vi "Ex 07 - C-Scan.vi"() -> ()   [LabVIEW 2026]
uses:
  <instrlib>/MicroPulse/Public/Data/Datatypes/MP - data formatting.ctl
  <instrlib>/MicroPulse/Public/Data/Datatypes/MP - amplitude reporting mode.ctl
  <instrlib>/MicroPulse/Public/Data/Datatypes/MP - averaging.ctl
  <instrlib>/MicroPulse/Public/Data/Datatypes/MP - transmit parameters.ctl
  <instrlib>/MicroPulse/Public/Data/Datatypes/MP - pulser voltage.ctl
  <instrlib>/MicroPulse/Public/Data/Datatypes/MP - pulse damping.ctl
  <instrlib>/MicroPulse/Public/Data/Datatypes/MP - test parameters.ctl
  <instrlib>/MicroPulse/Public/Data/Datatypes/MP - receive parameters.ctl
  <instrlib>/MicroPulse/Public/Data/Datatypes/MP - display gate.ctl
  <instrlib>/MicroPulse/Public/Data/Datatypes/MP - waveform type.ctl
  <instrlib>/MicroPulse/Public/Data/Datatypes/MP - analogue filter.ctl
  <instrlib>/MicroPulse/Public/Data/Datatypes/MP - frequency filter.ctl
  <instrlib>/MicroPulse/Public/Data/Datatypes/MP - digital filtering.ctl
  <instrlib>/MicroPulse/Public/Data/Datatypes/MP - high pass filter.ctl
  <instrlib>/MicroPulse/Public/Data/Datatypes/MP - low pass filter.ctl
  <instrlib>/MicroPulse/Public/Data/Datatypes/TCP config.ctl
  <instrlib>/MicroPulse/Public/Data/Datatypes/MP - multi-gate inspection.ctl
  <instrlib>/MicroPulse/Public/Data/Datatypes/MP - multigate inspection gate parameters.ctl
  <instrlib>/MicroPulse/Public/Data/Datatypes/MP - hysteresis level.ctl
  <instrlib>/MicroPulse/Public/Data/Datatypes/MP - multigate mode.ctl
  <instrlib>/MicroPulse/Public/Data/Datatypes/MP - echo gate parameters.ctl
  <instrlib>/MicroPulse/Public/Data/Datatypes/MP - echo gate mode.ctl
  <instrlib>/MicroPulse/Public/Data/Datatypes/MP - data output format.ctl
  <instrlib>/MicroPulse/Public/Data/Datatypes/MP - sample frequency.ctl
  <instrlib>/MicroPulse/Public/Data/Datatypes/MP - instrument type.ctl
  <instrlib>/MicroPulse/Public/Data/Datatypes/MP - fly scan range.ctl
  <instrlib>/MicroPulse/Public/Data/Datatypes/MP - inspection direction.ctl
  <instrlib>/MicroPulse/Public/Data/Datatypes/MP - encoder settings.ctl
  <instrlib>/MicroPulse/Public/Data/Datatypes/MP - encoder type.ctl
  <instrlib>/MicroPulse/Public/Data/Datatypes/MP - request system status.ctl
  <instrlib>/MicroPulse/Public/Data/Datatypes/MP - encoder mode.ctl
  <instrlib>/MicroPulse/Public/Data/Datatypes/PNDT - colour map selector.ctl
  <instrlib>/MicroPulse/Public/Data/Datatypes/MP - C-Scan Definition.ctl
  <instrlib>/MicroPulse/Public/Data/Datatypes/MP - fly scan range (timed).ctl
  <instrlib>/MicroPulse/Examples/SubVIs/Main Program State - Enum.ctl
  <instrlib>/MicroPulse/Public/Data/Datatypes/MP - fly inspection tests.ctl
  <instrlib>/MicroPulse/Public/Helper VIs/Low Level/FGV - B-Scan Active - Action [Enum].ctl
  <instrlib>/MicroPulse/Public/Helper VIs/Low Level/FGV - C-Scan Active - Action [Enum].ctl
  <vilib>/ErrorRing/Error Ring.xnode
  <instrlib>/MicroPulse/MicroPulse_Driver.lvlib
panel:
  in  "Scan definition":T1={"Max Scan Length"=100, "Update Rate"=100, "Direction"=enum."Forwards"} {"Update Rate" format="%#_6f"; "Max Scan Length" format="%#_6f"}
  out "C-Scan In Progress?":bool
  out "Y Current Position":dbl format="%#_6f mm"
  out "C-Scan Chart":u16[][](graph)
  in  "Centre Cursor":bool
  in  "Get Status":bool
  in  "Colour Map":T3
  out "B-Scan In Progress?":bool
  in  "Stop C-Scan":bool
  out "B-Scan Chart":u16[][](graph)
  in  "Request System Status":T4 caption="[STS]"
  out "X Current Position":dbl format="%#_6f mm"
  in  "Test Tab":T5(tab)
  in  "Data Formatting":T6={"Amplitude Mode"=enum."Peaks + Ascan for Multigate", "Averaging"=enum."None", "Coupling Level"=0} {"Coupling Level" max=4095 step=1}
  in  "Transmit Parameters":T9={"Pulse Voltage"=enum."50V", "Pulse Shape"={"Damping"=enum."660W", "Width"=250}} {"Pulse Shape"."Width" min=16 max=1010 step=50 format="%.0fns"}
  in  "Test Parameters":T12={"Test No."=1, "Tx Channel"=1, "Rx Channel"=1} {"Rx Channel" min=1 max=1024; "Tx Channel" min=1 max=1024}
  in  "Receive Parameters":T13={"Display Gate"={"Start"=0.0, "Length"=100.0}, "Delay"=0.0, "Waveform Type"=enum."Rectified Signal", "Gain"=50.0, "Analogue Filtering"={"Bandpass"=enum."No change", "Smoothing"=1}, "Digital Filtering"={"High Pass Filter"=enum."None", "Low Pass Filter"=enum."None"}} {"Delay" format="%#_g us"; "Display Gate"."Length" min=0.0 max=64000.0 step=1.0 format="%#_g us"; "Display Gate"."Start" min=0.0 max=64000.0 step=1.0 format="%#_g us"; "Analogue Filtering"."Smoothing" min=1 max=11 step=1; "Gain" min=-6.0 max=70.0 step=0.25 format="%.2fdB"}
  in  "Multi Gate Inspection":T21={"Gate 1"={"Start (us)"=15.0, "Length (us)"=50.0, "Threshold"=80, "Enabled?"=TRUE, "Max # Peaks"=8, "Hysteresis"=enum."6dB", "Mode"=enum."All Peaks In Gate", "Inverted?"=FALSE, "Colour "=16716306}, "Gate 2"={"Start (us)"=30.0, "Length (us)"=10.0, "Threshold"=50, "Enabled?"=FALSE, "Max # Peaks"=8, "Hysteresis"=enum."6dB", "Mode"=enum."All Peaks In Gate", "Inverted?"=FALSE, "Colour "=641024}, "Gate 3"={"Start (us)"=50.0, "Length (us)"=10.0, "Threshold"=30, "Enabled?"=FALSE, "Max # Peaks"=8, "Hysteresis"=enum."6dB", "Mode"=enum."All Peaks In Gate", "Inverted?"=FALSE, "Colour "=4532}, "Gate 4"={"Start (us)"=65.0, "Length (us)"=10.0, "Threshold"=10, "Enabled?"=FALSE, "Max # Peaks"=8, "Hysteresis"=enum."6dB", "Mode"=enum."All Peaks In Gate", "Inverted?"=FALSE, "Colour "=8978537}} {"Gate 4"."Max # Peaks" min=1 max=80 step=1; "Gate 4"."Threshold" min=10 step=10; "Gate 4"."Length (us)" min=0.0 max=96000.0 step=1.0; "Gate 4"."Start (us)" min=0.0 max=64000.0 step=1.0; "Gate 3"."Max # Peaks" min=1 max=80 step=1; "Gate 3"."Threshold" min=10 step=10; "Gate 3"."Length (us)" min=0.0 max=96000.0 step=1.0; "Gate 3"."Start (us)" min=0.0 max=64000.0 step=1.0; "Gate 2"."Max # Peaks" min=1 max=80 step=1; "Gate 2"."Threshold" min=10 step=10; "Gate 2"."Length (us)" min=0.0 max=96000.0 step=1.0; "Gate 2"."Start (us)" min=0.0 max=64000.0 step=1.0; "Gate 1"."Max # Peaks" min=1 max=80 step=1; "Gate 1"."Threshold" min=10 step=10; "Gate 1"."Length (us)" min=0.0 max=96000.0 step=1.0; "Gate 1"."Start (us)" min=0.0 max=64000.0 step=1.0}
  in  "Echo Gate Parameters":T25={"Start (us)"=10.0, "Length (us)"=20.0, "Threshold"=120, "Colour"=2731480} {"Threshold" min=10 max=4095 step=10; "Length (us)" min=0.0 max=96000.0 step=1.0; "Start (us)" min=0.0 max=64000.0 step=1.0}
  in  "Echo Gate Mode":T26
  in  "Set Position Y":bool
  in  "Position To Set Y":dbl caption="mm"
  in  "Encoder Reporting Mode":T27=enum."32-bit + LLC" caption="[ENCM]"
  in  "Set Position X":bool
  in  "Position To Set X":dbl caption="mm"
  in  "Encoder Settings":T28={"Encoder Type"=enum."Quadrature", "Counts/mm"=100, "Enable Termination?"=FALSE, "Multiplier"=2, "Backlash Period (s)"=10.0, "Encoder Filter"=0} {"Encoder Filter" max=255; "Backlash Period (s)" min=0.0005 max=10.0 step=0.0005; "Multiplier" min=1 max=100000; "Counts/mm" min=1 max=100000}
  in  "Axis No.":u8=1 min=1 max=4
  in  "Scan Choice":enum32{"Absolute Scan [FLX+FLZ]", "Free Scan"}(tab)
  in  "Axis 1 Scan":T30={"Scan Start"=0.0, "Scan Length"=80.0, "Inspection Resolution"=0.5, "Direction"=enum."Forwards"} caption="Primary Axis 1 Scan" {"Inspection Resolution" format="%#_6f"; "Scan Start" format="%#_6f"; "Scan Length" format="%#_6f"}
  in  "Start Test":bool
  in  "Axis 2 Scan":T31={"Index Start"=0.0, "Index Length"=10.0, "Indexing\nResolution"=1.0, "Ch1 Start"=0.0, "Ch1 Finish"=0.0, "Ch2 Start"=0.0, "Ch2 Finish"=0.0} caption="Secondary Axis 2 Scan" {"Ch2 Finish" format="%#_6f"; "Ch2 Start" format="%#_6f"; "Ch1 Finish" format="%#_6f"; "Ch1 Start" format="%#_6f"; "Index Start" format="%#_6f"; "Index Length" format="%#_6f"; "Indexing\nResolution" format="%#_6f"}
  in  "FreeScan PRF":u16=1000 caption="[PRF]" min=1 max=20000 step=100 format="%dHz"
  in  "Y Scan definition":T32={"Max Y Scan Length"=100.0, "Indexing\nResolution"=1.0, "Ch1 Start"=0.0, "Ch1 Finish"=0.0, "Ch2 Start"=0.0, "Ch2 Finish"=0.0} {"Ch2 Finish" format="%#_6f"; "Ch2 Start" format="%#_6f"; "Ch1 Finish" format="%#_6f"; "Ch1 Start" format="%#_6f"; "Max Y Scan Length" format="%#_6f"; "Indexing\nResolution" format="%#_6f"}
  out "Scan Timer Enabled?":bool
  in  "Start Free Scan":bool
  in  "X Scan definition":T33={"Max X Scan Length"=100, "Indexing\nResolution"=1} {"Indexing\nResolution" format="%#_6f"; "Max X Scan Length" format="%#_6f"}
  out "Instrument Type":T34
  out "Sample Frequency out":T35 caption="Sample Frequency"
  out "Stop":bool
  in  "Sample Frequency":T35
  in  "PRF":u16=20000 caption="[PRF]" min=1 max=20000 step=100 format="%dHz"
  in  "Data Output Format":T36=enum."8-bit Mode" caption="[DOF]"
  in  "Gate No.":i32=1
  out "peak data":cluster{"Time":dbl[], "Level":u16[]} {"Time" format="%_6g"}
  out "A-Scan + Peaks":cluster{"timebase":dbl[], "data":u16[]}[](graph) caption="A-Scan + Peaks Test 1"
  in  "Acquire Single Scan":bool
  in  "Stop Acquisition":bool
  in  "Start Acquisition":bool
  out "Command List":string
  in  "QUIT":bool
  out "running average PRF":dbl format="%0.2f"
  out "live error out":errorcluster
  out "message count":i32
  out "System Messages":string
  in  "TCP config":T37={"Connection ID"=refnum, "IP address"="10.1.1.2", "host port"=1067, "OC timeout"=5000, "Read timeout"=2000, "Write timeout"=100} {"Write timeout" format="%dms"; "Read timeout" format="%dms"; "OC timeout" format="%dms"}
  # "Example 07 - C-Scans\n\nSet all controls to the required values\nbefore running the Test.\n\nWhile running, test parameters may NOT be  changed, though gate and UT parameters may."
  # "For this example, the Encoder Settings will be the same for both axes."
  # "Set Current Position X"
  # "Set Current Position Y"
  # "C-Scan Index"
  # "Y-Scan Index"
  # "X-Scan Index"
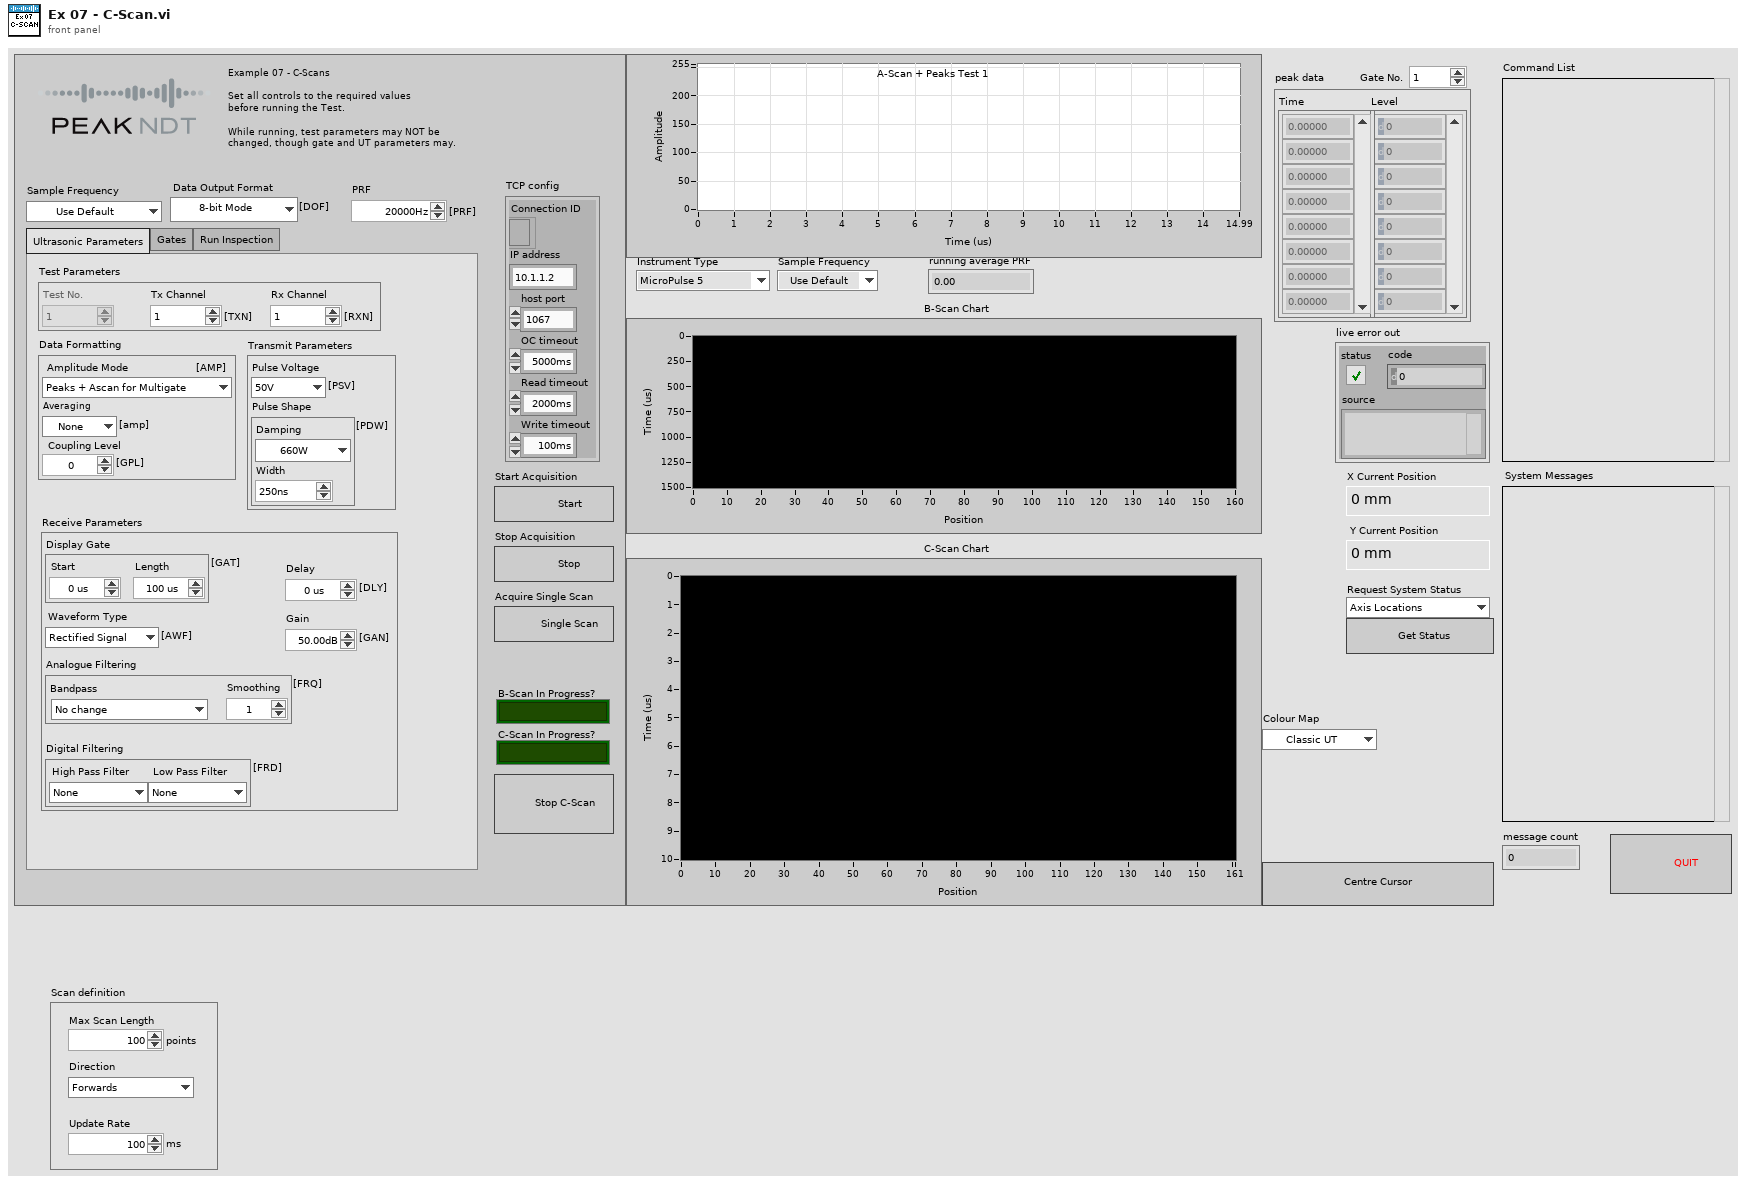
[diagram p1: front panel]
types:
  T1 = typedef "MicroPulse_Driver.lvlib/MP - fly scan range (timed).ctl" = cluster{"Max Scan Length":i32, "Update Rate":i32, "Direction":T2}
  T2 = typedef "MicroPulse_Driver.lvlib/MP - inspection direction.ctl" = enum16{"Forwards", "Backwards"}
  T3 = typedef "MicroPulse_Driver.lvlib/PNDT - colour map selector.ctl" = enum16{"Classic UT", "Ultrasonic", "Inverse Grey", "Grey Scale", "TOFD", "Fire", "Rainbow", "Ice", "Original"}
  T4 = typedef "MicroPulse_Driver.lvlib/MP - request system status.ctl" = enum16{"Axis Locations", "MPE settings", "BKL settings", "SPA settings", "I/O status", "RST elapsed time", "System Status", "Temperatures", "System Log", "Erase system Log", "RST message", "Master System Msg", "Slave System Msg"}
  T5 = enum32{"Ultrasonic Parameters", "Gates", "Run Inspection"}
  T6 = typedef "MicroPulse_Driver.lvlib/MP - data formatting.ctl" = cluster{"Amplitude Mode":T7, "Averaging":T8, "Coupling Level":u32}
  T7 = typedef "MicroPulse_Driver.lvlib/MP - amplitude reporting mode.ctl" = enum16{"1st Peak in gate", "Maximum Peak in gate", "All Peaks", "Ascan Data", "1st Threshold Crossing Peak", "Ascan + Peaks", "All Peaks for Multigate", "Peaks + Ascan for Multigate", "Peaks + P_Ascan for Multigate", "Full Matrix Capture"}
  T8 = typedef "MicroPulse_Driver.lvlib/MP - averaging.ctl" = enum16{"None", "2", "4", "8", "16", "32", "64", "128", "256"}
  T9 = typedef "MicroPulse_Driver.lvlib/MP - transmit parameters.ctl" = cluster{"Pulse Voltage":T10, "Pulse Shape":cluster{"Damping":T11, "Width":u32}}
  T10 = typedef "MicroPulse_Driver.lvlib/MP - pulser voltage.ctl" = enum16{"50V", "100V", "150V", "200V", "250V", "300V"}
  T11 = typedef "MicroPulse_Driver.lvlib/MP - pulse damping.ctl" = enum16{"660W", "458W", "220W", "149W", "102W", "82W", "63W", "51W"}
  T12 = typedef "MicroPulse_Driver.lvlib/MP - test parameters.ctl" = cluster{"Test No.":u32, "Tx Channel":u32, "Rx Channel":u32}
  T13 = typedef "MicroPulse_Driver.lvlib/MP - receive parameters.ctl" = cluster{"Display Gate":T14, "Delay":dbl, "Waveform Type":T15, "Gain":dbl, "Analogue Filtering":T16, "Digital Filtering":T18}
  T14 = typedef "MicroPulse_Driver.lvlib/MP - display gate.ctl" = cluster{"Start":dbl, "Length":dbl}
  T15 = typedef "MicroPulse_Driver.lvlib/MP - waveform type.ctl" = enum16{"Rectified Signal", "RF Signal", "+Half Wave", "-Half Wave"}
  T16 = typedef "MicroPulse_Driver.lvlib/MP - analogue filter.ctl" = cluster{"Bandpass":T17, "Smoothing":u16}
  T17 = typedef "MicroPulse_Driver.lvlib/MP - frequency filter.ctl" = enum16{"No change", "1MHz Bandpass", "2MHz Bandpass", "4MHz Bandpass", "5MHz Bandpass", "10MHz Bandpass", "2.5-18MHz Broadband", "0.75-12MHz  Broadband", "0.5MHz Bandpass", "5MHz 2nd Order TOFD", "10MHz 2nd Order TOFD", "3.0-25MHz Broadband", "3.0-30MHz Broadband"}
  T18 = typedef "MicroPulse_Driver.lvlib/MP - digital filtering.ctl" = cluster{"High Pass Filter":T19, "Low Pass Filter":T20}
  T19 = typedef "MicroPulse_Driver.lvlib/MP - high pass filter.ctl" = enum16{"None", "0.7MHz", "1.5MHz", "4.0MHz", "7.5MHz", "10.0MHz", "User Defined"}
  T20 = typedef "MicroPulse_Driver.lvlib/MP - low pass filter.ctl" = enum16{"None", "1.8MHz", "3.0MHz", "6.0MHz", "8.0MHz", "12.0MHz", "User Defined"}
  T21 = typedef "MicroPulse_Driver.lvlib/MP - multi-gate inspection.ctl" = cluster{"Gate 1":T22, "Gate 2":T22, "Gate 3":T22, "Gate 4":T22}
  T22 = typedef "MicroPulse_Driver.lvlib/MP - multigate inspection gate parameters.ctl" = cluster{"Start (us)":dbl, "Length (us)":dbl, "Threshold":u16, "Enabled?":bool, "Max # Peaks":u16, "Hysteresis":T23, "Mode":T24, "Inverted?":bool, "Colour ":u32}
  T23 = typedef "MicroPulse_Driver.lvlib/MP - hysteresis level.ctl" = enum16{"None", "3dB", "6dB", "9dB", "12dB"}
  T24 = typedef "MicroPulse_Driver.lvlib/MP - multigate mode.ctl" = enum16{"1st Peak in Gate", "Largest Peak In Gate", "All Peaks In Gate", "1st Threshold Crossing"}
  T25 = typedef "MicroPulse_Driver.lvlib/MP - echo gate parameters.ctl" = cluster{"Start (us)":dbl, "Length (us)":dbl, "Threshold":u16, "Colour":u32}
  T26 = typedef "MicroPulse_Driver.lvlib/MP - echo gate mode.ctl" = enum16{"Echo Trigger OFF", "Echo Gate Display Mode", "Echo Trigger ON", "Multi Gate or FMC Mode", "Reserved", "PA - Echo Trigger ON"}
  T27 = typedef "MicroPulse_Driver.lvlib/MP - encoder mode.ctl" = enum16{"24-bit + LCI", "32-bit + LCI", "32-bit + LLC", "24-bit + STS6", "32-bit + STS6", "32-bit + LLC+STS6"}
  T28 = typedef "MicroPulse_Driver.lvlib/MP - encoder settings.ctl" = cluster{"Encoder Type":T29, "Counts/mm":u32, "Enable Termination?":bool, "Multiplier":u32, "Backlash Period (s)":dbl, "Encoder Filter":u32}
  T29 = typedef "MicroPulse_Driver.lvlib/MP - encoder type.ctl" = enum16{"Quadrature", "Step/Direction"}
  T30 = typedef "MicroPulse_Driver.lvlib/MP - fly scan range.ctl" = cluster{"Scan Start":dbl, "Scan Length":dbl, "Inspection Resolution":dbl, "Direction":T2}
  T31 = typedef "MicroPulse_Driver.lvlib/MP - C-Scan Definition.ctl" = cluster{"Index Start":dbl, "Index Length":dbl, "Indexing\nResolution":dbl, "Ch1 Start":dbl, "Ch1 Finish":dbl, "Ch2 Start":dbl, "Ch2 Finish":dbl}
  T32 = cluster{"Max Y Scan Length":dbl, "Indexing\nResolution":dbl, "Ch1 Start":dbl, "Ch1 Finish":dbl, "Ch2 Start":dbl, "Ch2 Finish":dbl}
  T33 = cluster{"Max X Scan Length":i32, "Indexing\nResolution":i32}
  T34 = typedef "MicroPulse_Driver.lvlib/MP - instrument type.ctl" = enum16{"MicroPulse 5", "LT1", "LT2", "LTPA", "MPLT", "MicroPulse 6", "PipeScanner", "<MicroPulse>", "Micropulse 4", "Simulated Data"}
  T35 = typedef "MicroPulse_Driver.lvlib/MP - sample frequency.ctl" = enum16{"Use Default", "200MHz (LT2 only)", "100MHz", "50MHz", "25MHz", "10MHz"}
  T36 = typedef "MicroPulse_Driver.lvlib/MP - data output format.ctl" = enum16{"", "8-bit Mode", "10-bit Mode", "12-bit Mode", "16-bit Mode", "8-bit Log Mode", "12-bit Packed Mode"}
  T37 = typedef "MicroPulse_Driver.lvlib/TCP config.ctl" = cluster{"Connection ID":refnum<k5>, "IP address":string, "host port":u16, "OC timeout":i32, "Read timeout":i32, "Write timeout":i32}
  T38 = typedef "Main Program State - Enum.ctl" = enum16{"Initialise", "Init HW", "Run", "Reset HW", "Shutdown"}
  T39 = typedef "MicroPulse_Driver.lvlib/FGV - B-Scan Active - Action [Enum].ctl" = enum16{"Read", "Read & Reset Start Flag", "Start B-Scan", "B-Scan Finished"}
  T40 = typedef "MicroPulse_Driver.lvlib/FGV - C-Scan Active - Action [Enum].ctl" = enum16{"Read", "Read & Reset Start Flag", "Start C-Scan", "C-Scan Finished"}
  T41 = typedef "MicroPulse_Driver.lvlib/MP - fly inspection tests.ctl" = enum16{"Conventional Tests", "Conv >> PA Tests", "PA >> Conv Tests", "PA Tests", "Group Tests", "PA Sweep as per FDEF"}
  T42 = typedef "MicroPulse_Driver.lvlib/MP-Registry Data-Cluster.ctl" = cluster{"Instrument Type":T34, "Serial #":u64, "Sample Frequency":T35, "dt (us)":dbl, "DOF":T36, "Material Velocity":dbl, "Asynch Reads":T43, "NUM of Tests":u32, "System Details":T44, "Gates":T46[], "Encoders":T28[], "CMD LUT":variant, "Command List":string}
  T43 = typedef "MicroPulse_Driver.lvlib/MP - asynch read mode.ctl" = enum16{"Disabled", "Enabled"}
  T44 = typedef "MicroPulse_Driver.lvlib/MP - general system status.ctl" = cluster{"System Type":T34, "Serial No.":u64, "Channels":cluster{"Conv":u8, "PA":u16, "Extra":u32}, "Sample Frequency":cluster{"Default":u8, "Actual":u8}, "Software Versions":string, "Data Output Format":cluster{"Default":T36, "Actual":T36}, "Temperatures":cluster{"System":u8, "Processor":u8, "Slave Sys":u8, "Slave Proc":u8}, "Tx Buffer Size":u32, "System Error":string, "No. of Cards":u8, "DAC Gain":i16, "Uptimes":cluster{"since Power":u32, "since RSTS":u32, "since SRST":u32}, "Voltages":cluster{"Nominal":dbl, "Measured":dbl, "Difference":dbl}[], "Interface Cards":T45[]}
  T45 = typedef "MicroPulse_Driver.lvlib/MP - interface card status.ctl" = cluster{"Status":u8, "Map":u8, "Board - T":u8, "FPGA - T":u8, "PAIF Status":string, "Version":string}
  T46 = typedef "MicroPulse_Driver.lvlib/MP - Registry Gates.ctl" = cluster{"Display Gate":T14, "ETM Mode":T26, "Echo Gate":T25, "Insp Gates":T22[]}
  T47 = typedef "LVPointDoubleTypeDef.ctl" = cluster{"Cursor X":dbl, "Cursor Y":dbl}
  T48 = typedef "LVBoundsTypeDef.ctl" = cluster{"Width":u32, "Height":u32}
  T49 = typedef "MicroPulse_Driver.lvlib/MP - scan data info.ctl" = cluster{"Message Header":u16, "Error Message":u16, "Test No.":u32, "Channel No.":u8, "Sweep No.":u32, "Gate No.":u32, "DOF":T36, "retain data":T50, "scan data":u16[], "scan length":i32, "scan index":i32, "peak data":cluster{"timebase":u16[], "data":u16[]}, "#peaks":i32, "PRF":dbl, "IP":cluster{"Axis No.":u8, "Location":u32, "MIP location":u32, "MIP?":bool}, "echo range":u16, "ETG":bool, "CAL 0 complete":bool, "Axis Positions":T51}
  T50 = typedef "MicroPulse_Driver.lvlib/MP - retain scan.ctl" = enum16{"None", "Ascan", "Peaks"}
  T51 = typedef "MicroPulse_Driver.lvlib/MP - axis positions (LLC).ctl" = cluster{"Axis 1":u32, "Axis 2":u32, "Axis 3":u32, "Axis 4":u32, "Status":u8}
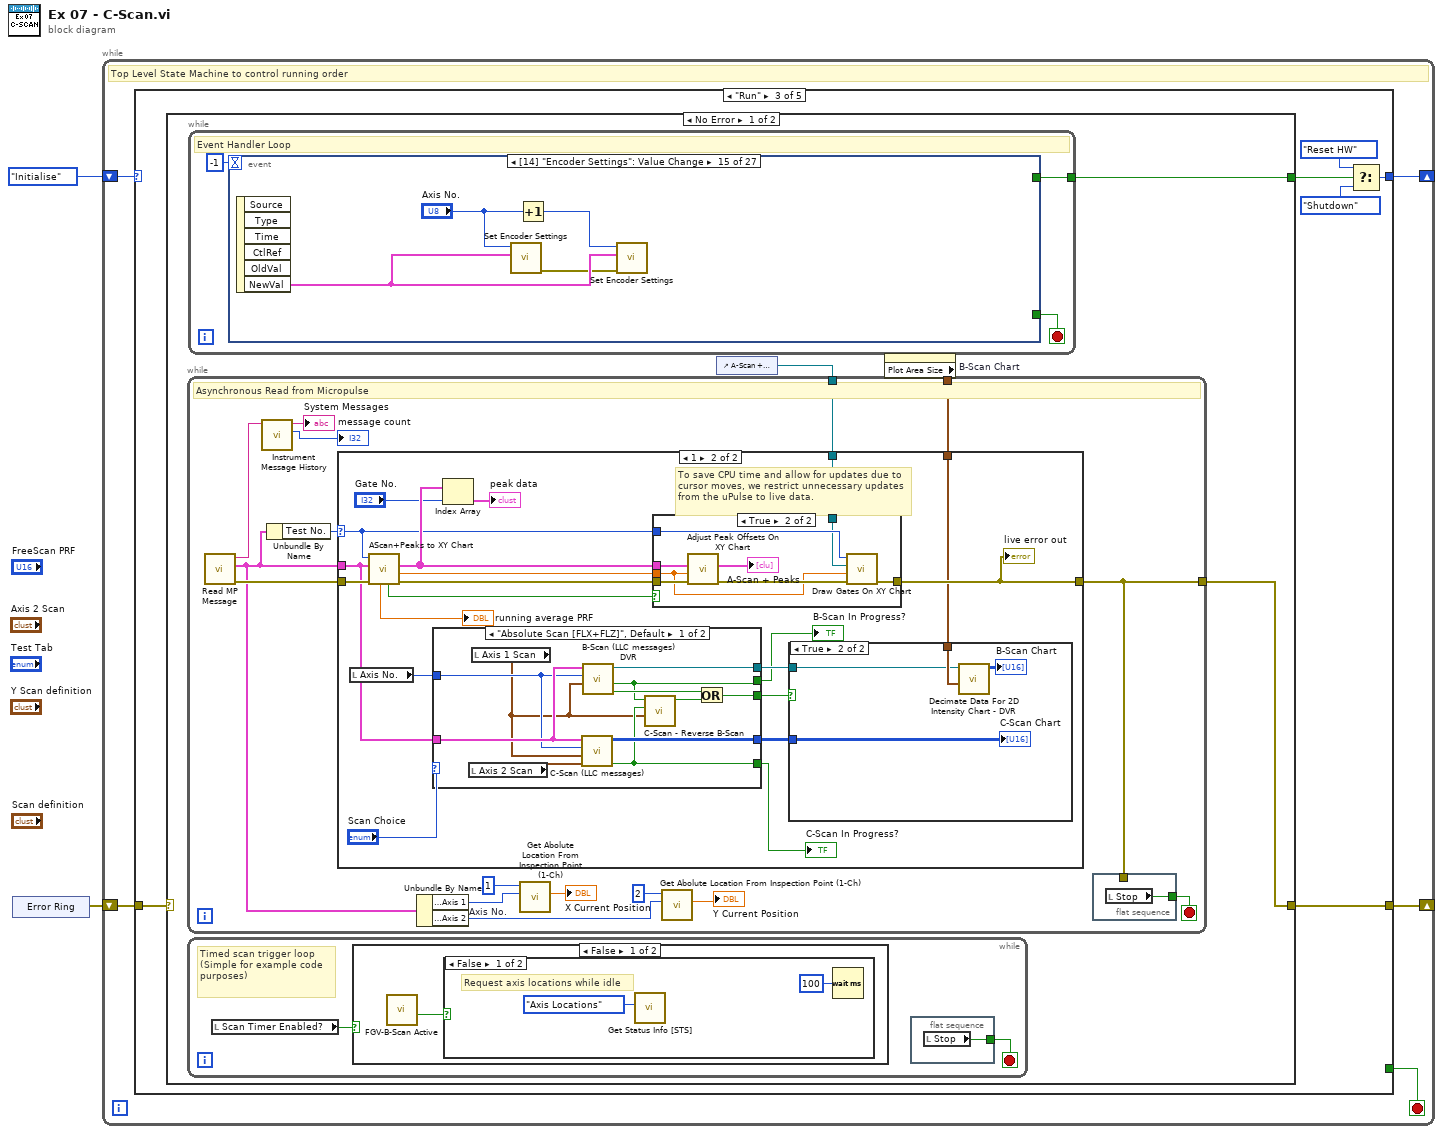
[diagram p0: block diagram]
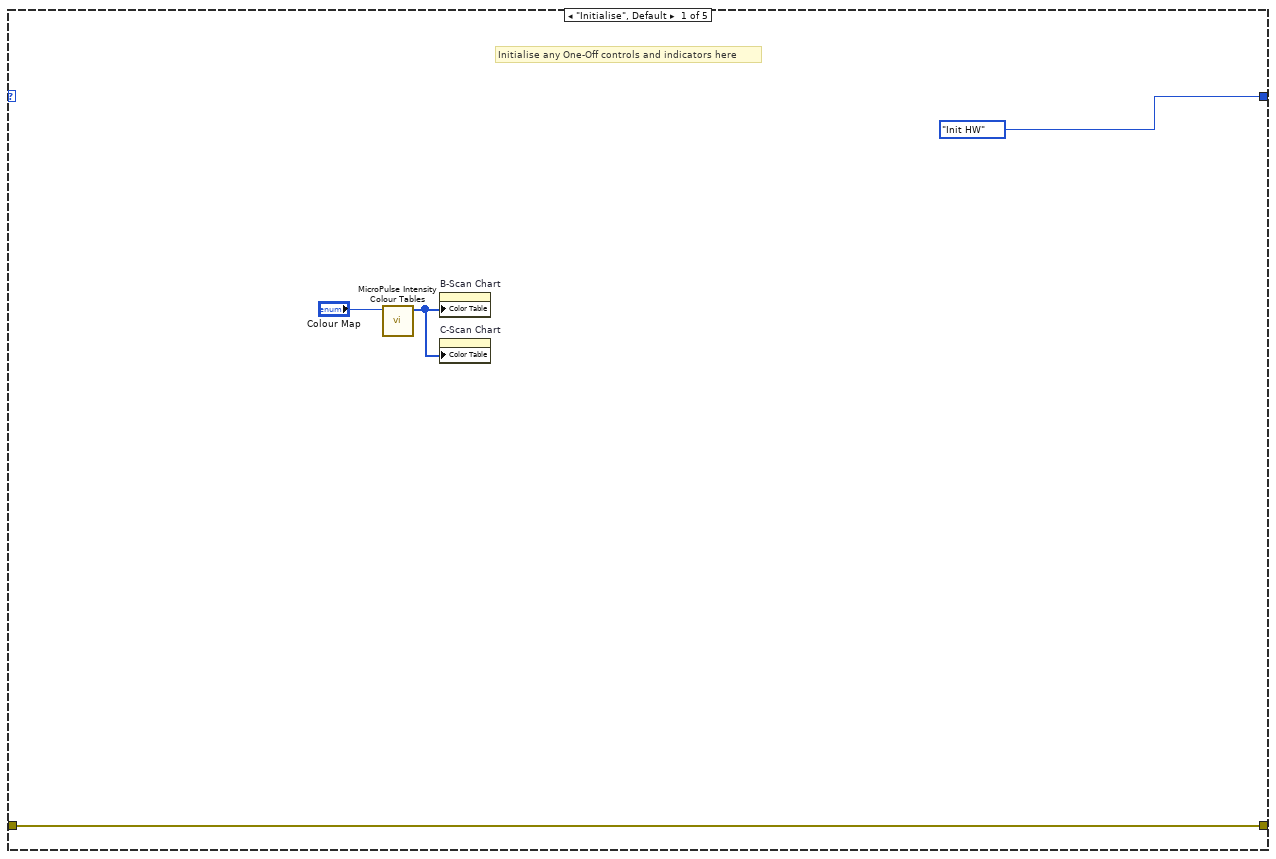
[diagram p2: hidden frame]
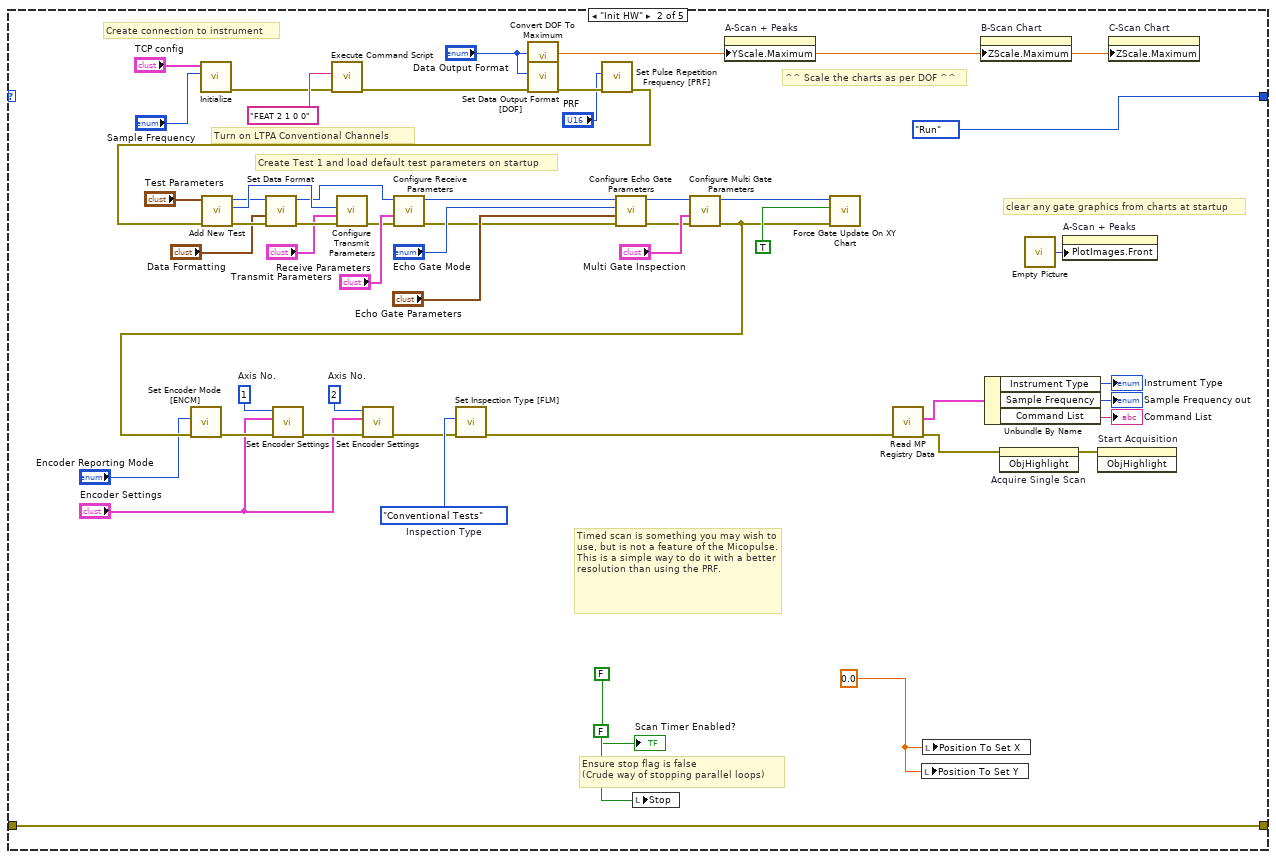
[diagram p3: hidden frame]
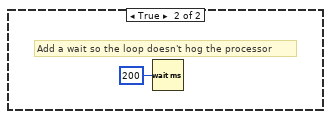
[diagram p4: hidden frame]
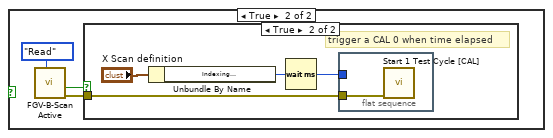
[diagram p5: hidden frame]
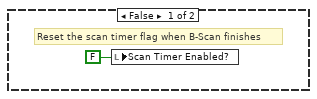
[diagram p6: hidden frame]
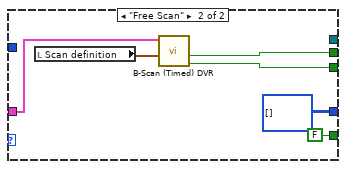
[diagram p10: hidden frame]
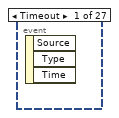
[diagram p11: hidden frame]
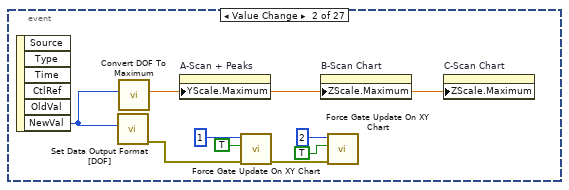
[diagram p12: hidden frame]
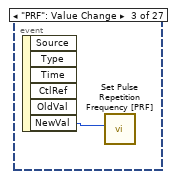
[diagram p13: hidden frame]
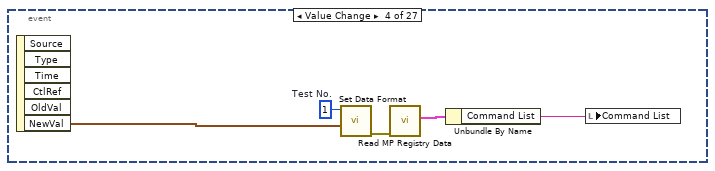
[diagram p14: hidden frame]
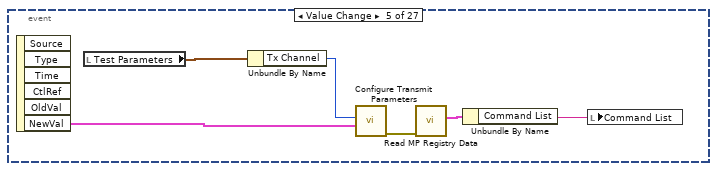
[diagram p15: hidden frame]
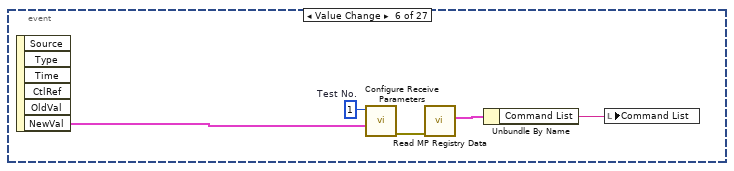
[diagram p16: hidden frame]
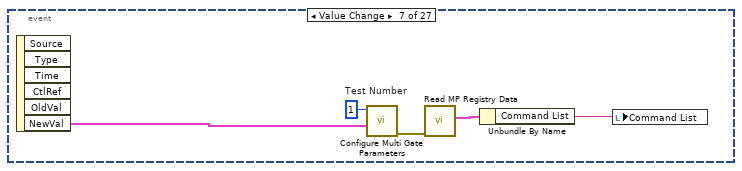
[diagram p17: hidden frame]
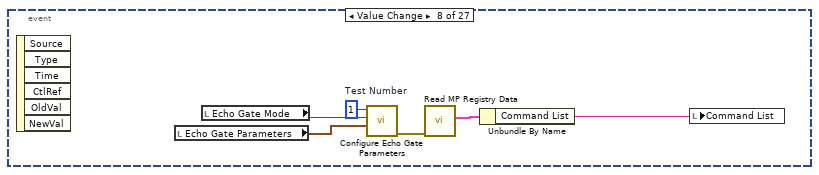
[diagram p18: hidden frame]
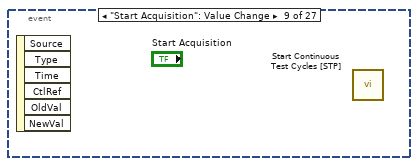
[diagram p19: hidden frame]
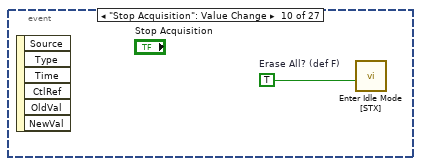
[diagram p20: hidden frame]
diagram:
  n1 = xnode "Error Ring"() -> ("error out"=w2:errorcluster)
  n2 = while {
    shift-right: [w4] -> _
    shift-left: Main_Program_State_-_Enum."Initialise" -> [w7]
    shift-right: [w5] -> _
    shift-left: w2 -> [w6]
    stop <- w3 stop-if-true
    # "Top Level State Machine to control running order"
    n3 = case shown="\"Run\"" w7 {
      tunnel: w6 -> [w10 w40 w68 w279 w284]
      tunnel: [w10 w40 w67 w278 w284] -> w5
      tunnel: [Main_Program_State_-_Enum."Init HW" Main_Program_State_-_Enum."Run" w63 Main_Program_State_-_Enum."Init HW" Main_Program_State_-_Enum."Initialise"] -> w4
      tunnel: [_ _ _ _ TRUE] -> w3
      frame "Initialise", Default {
        # "Initialise any One-Off controls and indicators here"
        n4 = call <instrlib>:"MicroPulse Intensity Colour Tables.vi"("Colour Map Type"="Colour Map") -> ("Colour Table"=w8:u32[])  [unwired: 10 in]
        n5 = property on="B-Scan Chart" class="IntGraph (strict)"("Color Table"=w8) -> ()  [unwired: 2 in, 2 out]
        n6 = property on="C-Scan Chart" class="IntGraph (strict)"("Color Table"=w8) -> ()  [unwired: 2 in, 2 out]
      }
      frame "Init HW" {
        w18 = u8 2  # Axis No.
        w19 = 0.0 ("Position To Set X")
        w22 = MP_-_fly_inspection_tests."Conventional Tests"  # Inspection Type
        w24 = u8 1  # Axis No.
        # "Turn on LTPA Conventional Channels"
        # "Timed scan is something you may wish to use, but is not a feature of the Micopulse.\nThis is a simple way to do it with a better resolution than using the PRF."
        # "^^ Scale the charts as per DOF ^^"
        # "Ensure stop flag is false\n(Crude way of stopping parallel loops)"
        # "Create connection to instrument"
        # "clear any gate graphics from charts at startup"
        # "Create Test 1 and load default test parameters on startup"
        n7 = call <instrlib>:"Initialize.vi"("Sample Frequency"="Sample Frequency", "TCP config"="TCP config") -> ("error out"=w13:errorcluster)  [unwired: 8 in, 1 out]
        n8 = call <instrlib>:"Execute Command Script.vi"("error in (no error)"=w13, "String in"="FEAT 2 1 0 0") -> ("error out"=w12:errorcluster)  [unwired: 7 in, 2 out]
        n9 = call <instrlib>:"Convert DOF To Maximum.vi"("Data Output Format"="Data Output Format") -> ("Data Maximum"=w20:dbl)  [unwired: 10 in]
        n10 = call <instrlib>:"Set Data Output Format [DOF].vi"("error in (no error)"=w12, "Mode"="Data Output Format") -> ("error out"=w33:errorcluster)  [unwired: 8 in, 1 out]
        n11 = call <instrlib>:"Set Pulse Repetition Frequency [PRF].vi"("error in (no error)"=w33, "Frequency (Hz)"="PRF") -> ("error out"=w31:errorcluster)  [unwired: 8 in, 1 out]
        n12 = call <instrlib>:"Add New Test.vi"("error in (no error)"=w31, "Test Parameters"="Test Parameters") -> ("error out"=w55:errorcluster, "Tx Channel out"=w54:u32, "Test No. out"=w50:u32)  [unwired: 6 in, 1 out]
        n13 = call <instrlib>:"Set Data Format.vi"("error in (no error)"=w55, "Data Formatting"="Data Formatting", "Test No."=w50) -> ("error out"=w45:errorcluster, "Test No. out"=w52:u32)  [unwired: 6 in, 1 out]
        n14 = call <instrlib>:"Configure Transmit Parameters.vi"("error in (no error)"=w45, "Transmit Parameters"="Transmit Parameters", "Tx Channel"=w54) -> ("error out"=w44:errorcluster)  [unwired: 7 in, 1 out]
        n15 = call <instrlib>:"Configure Receive Parameters.vi"("error in (no error)"=w44, "Receive Parameters"="Receive Parameters", "Test No."=w52) -> ("error out"=w46:errorcluster, "Test No. out"=w51:u32)  [unwired: 6 in, 1 out]
        n16 = call <instrlib>:"Configure Echo Gate Parameters.vi"("error in (no error)"=w46, "Echo Gate Parameters"="Echo Gate Parameters", "Echo Trigger Mode"="Echo Gate Mode", "Test Number"=w51) -> ("error out"=w48:errorcluster, "Test Number Out"=w53:u32)  [unwired: 5 in, 1 out]
        n17 = local write "Stop"(FALSE ("stop")) -> ()
        n18 = call <instrlib>:"Configure Multi Gate Parameters.vi"("error in (no error)"=w48, "Multi Gate Inspection"="Multi Gate Inspection", "Test Number"=w53) -> ("error out"=w27:errorcluster, "Test Number out"=w38:u32)  [unwired: 6 in, 1 out]
        n19 = call <instrlib>:"Set Encoder Mode [ENCM].vi"("error in (no error)"=w27, "Encoder Mode"="Encoder Reporting Mode") -> ("error out"=w25:errorcluster)  [unwired: 8 in, 1 out]
        n20 = call <instrlib>:"Set Encoder Settings.vi"("error in (no error)"=w25, "Encoder Settings"="Encoder Settings", "Axis No."=w24) -> ("error out"=w17:errorcluster)  [unwired: 8 in]
        n21 = call <instrlib>:"Set Encoder Settings.vi"("error in (no error)"=w17, "Encoder Settings"="Encoder Settings", "Axis No."=w18) -> ("error out"=w16:errorcluster)  [unwired: 8 in]
        n22 = call <instrlib>:"Set Inspection Type [FLM].vi"("error in (no error)"=w16, "Inspection Type"=w22) -> ("error out"=w23:errorcluster)  [unwired: 8 in, 1 out]
        n23 = property on="A-Scan + Peaks" class="XYGraph (strict)"("YScale.Maximum"=w20) -> ()  [unwired: 2 in, 2 out]
        n24 = call <instrlib>:"Force Gate Update On XY Chart.vi"("error in (no error)"=w27, "Set?"=TRUE, "Test No."=w38) -> ()  [unwired: 6 in, 3 out]
        n25 = call <instrlib>:"Read MP Registry Data.vi"("error in (no error)"=w23) -> ("error out"=w61:errorcluster, "Micropulse Data"=w59:T42)  [unwired: 7 in, 2 out]
        n26 = local write "Position To Set Y"(w19) -> ()
        n27 = local write "Position To Set X"(w19) -> ()
        n28 = property on="B-Scan Chart" class="IntGraph (strict)"("ZScale.Maximum"=w20) -> ()  [unwired: 2 in, 2 out]
        n29 = Unbundle By Name(w59) -> ("Instrument Type"=→"Instrument Type":T34, "Sample Frequency"=→"Sample Frequency out":T35, "Command List"=→"Command List":string)
        n30 = invoke on="Acquire Single Scan" class="Bool" method="ObjHighlight"(error in=w61) -> (error out=w62:errorcluster)  [unwired: 2 in, 2 out]
        n31 = call "Empty Picture"() -> ("empty picture"=w39:picture)
        n32 = property on="A-Scan + Peaks" class="XYGraph (strict)"("PlotImages.Front"=w39) -> ()  [unwired: 2 in, 2 out]
        n33 = invoke on="Start Acquisition" class="Bool" method="ObjHighlight"(error in=w62) -> ()  [unwired: 2 in, 3 out]
        n34 = property on="C-Scan Chart" class="IntGraph (strict)"("ZScale.Maximum"=w20) -> ()  [unwired: 2 in, 2 out]
        "Scan Timer Enabled?" <- FALSE ("Scan Timer Enabled?")
      }
      frame "Run" {
        n35 = case shown="No Error" w68 {
          selector: w68 -> [_ w277]
          tunnel: [w71 w277] -> w67
          tunnel: [w70 FALSE] -> w64
          frame No Error {
            n36 = while {
              stop <- w73 stop-if-true
              # "Timed scan trigger loop\n(Simple for example code purposes)"
              n37 = local read "Scan Timer Enabled?"() -> (w74:bool)
              n38 = case shown="False" w74 {
                frame False {
                  n39 = call <instrlib>:"FGV-B-Scan Active.vi"() -> ("B-Scan In Progress?"=w76:bool)  [unwired: 9 in, 2 out]
                  n40 = case shown="False" w76 {
                    frame False {
                      # "Request axis locations while idle"
                      n41 = call <instrlib>:"Get Status Info [STS].vi"("Request System Status"=MP_-_request_system_status."Axis Locations") -> ()  [unwired: 9 in, 2 out]
                      n42 = Wait (ms)(milliseconds to wait=u32 100) -> ()  [unwired: 1 out]
                    }
                    frame True {
                      # "Add a wait so the loop doesn't hog the processor"
                      n43 = Wait (ms)(milliseconds to wait=u32 200) -> ()  [unwired: 1 out]
                    }
                  }
                }
                frame True {
                  n44 = call <instrlib>:"FGV-B-Scan Active.vi"("Action"=FGV_-_B-Scan_Active_-_Action_[Enum]."Read") -> ("error out"=w80:errorcluster, "B-Scan In Progress?"=w81:bool)  [unwired: 8 in, 1 out]
                  n45 = case shown="True" w81 {
                    tunnel: w80 -> [_ w84]
                    frame False {
                      # "Reset the scan timer flag when B-Scan finishes"
                      n46 = local write "Scan Timer Enabled?"(FALSE ("Scan Timer Enabled?")) -> ()
                    }
                    frame True {
                      # "trigger a CAL 0 when time elapsed"
                      n47 = Unbundle By Name("X Scan definition") -> ("Indexing\nResolution"=w86:i32)
                      n48 = Wait (ms)(milliseconds to wait=w86) -> (millisecond timer value=w85:u32)
                      n49 = flat-sequence {
                        tunnel: w85 -> [_]
                        tunnel: w84 -> [w88]
                        frame #0 {
                          n50 = call <instrlib>:"Start 1 Test Cycle [CAL].vi"("error in (no error)"=w88) -> ()  [unwired: 9 in, 2 out]
                        }
                      }
                    }
                  }
                }
              }
              n51 = flat-sequence {
                tunnel: [w75] -> w73
                frame #0 {
                  n52 = local read "Stop"() -> (w75:bool)
                }
              }
            }
            n53 = while {
              tunnel: [w158] -> w70
              stop <- w159 stop-if-true
              # "Event Handler Loop"
              n54 = event shown="[14] \"Encoder Settings\": Value Change" {
                selector: _ -> [_ _ _ _ _ _ _ _ _ _ _ _ _ _ _ _ _ _ _ _ _ _ _ _ _ _ _]
                dyn-events: _ -> [_ _ _ _ _ _ _ _ _ _ _ _ _ _ _ _ _ _ _ _ _ _ _ _ _ _ _]
                timeout: -1 -> [_ _ _ _ _ _ _ _ _ _ _ _ _ _ _ _ _ _ _ _ _ _ _ _ _ _ _]
                tunnel: [_ _ _ _ _ _ _ _ _ _ _ _ w199 _ _ _ _ _ _ _ _ _ _ _ _ _ TRUE ("stop")] -> w159
                tunnel: [_ _ _ _ _ _ _ _ _ _ _ _ TRUE _ _ _ _ _ _ _ _ _ _ _ _ FALSE _] -> w158
                event Timeout {
                  n55 = event-data() -> ()  [unwired: 1 in, 3 out]
                }
                event Value Change {
                  n56 = event-data() -> ("NewVal"=w161:T36)  [unwired: 1 in, 5 out]
                  n57 = call <instrlib>:"Set Data Output Format [DOF].vi"("Mode"=w161) -> ("error out"=w163:errorcluster)  [unwired: 9 in, 1 out]
                  n58 = call <instrlib>:"Convert DOF To Maximum.vi"("Data Output Format"=w161) -> ("Data Maximum"=w160:dbl)  [unwired: 10 in]
                  n59 = property on="A-Scan + Peaks" class="XYGraph (strict)"("YScale.Maximum"=w160) -> ()  [unwired: 2 in, 2 out]
                  n60 = call <instrlib>:"Force Gate Update On XY Chart.vi"("error in (no error)"=w163, "Set?"=TRUE, "Test No."=u32 1) -> ("error out"=w162:errorcluster)  [unwired: 6 in, 2 out]
                  n61 = property on="B-Scan Chart" class="IntGraph (strict)"("ZScale.Maximum"=w160) -> ()  [unwired: 2 in, 2 out]
                  n62 = call <instrlib>:"Force Gate Update On XY Chart.vi"("error in (no error)"=w162, "Set?"=TRUE, "Test No."=u32 2) -> ()  [unwired: 6 in, 3 out]
                  n63 = property on="C-Scan Chart" class="IntGraph (strict)"("ZScale.Maximum"=w160) -> ()  [unwired: 2 in, 2 out]
                }
                event "PRF": Value Change {
                  n64 = event-data() -> ("NewVal"=w168:u16)  [unwired: 1 in, 5 out]
                  n65 = call <instrlib>:"Set Pulse Repetition Frequency [PRF].vi"("Frequency (Hz)"=w168) -> ()  [unwired: 9 in, 2 out]
                }
                event Value Change {
                  w170 = u32 1  # Test No.
                  n66 = event-data() -> ("NewVal"=w169:T6)  [unwired: 1 in, 5 out]
                  n67 = call <instrlib>:"Set Data Format.vi"("Data Formatting"=w169, "Test No."=w170) -> ("error out"=w173:errorcluster)  [unwired: 7 in, 2 out]
                  n68 = call <instrlib>:"Read MP Registry Data.vi"("error in (no error)"=w173) -> ("Micropulse Data"=w172:T42)  [unwired: 7 in, 3 out]
                  n69 = Unbundle By Name(w172) -> ("Command List"=w171:string)
                  n70 = local write "Command List"(w171) -> ()
                }
                event Value Change {
                  n71 = event-data() -> ("NewVal"=w178:T9)  [unwired: 1 in, 5 out]
                  n72 = local read "Test Parameters"() -> (w179:T12)
                  n73 = Unbundle By Name(w179) -> ("Tx Channel"=w177:u32)
                  n74 = call <instrlib>:"Configure Transmit Parameters.vi"("Transmit Parameters"=w178, "Tx Channel"=w177) -> ("error out"=w175:errorcluster)  [unwired: 8 in, 1 out]
                  n75 = call <instrlib>:"Read MP Registry Data.vi"("error in (no error)"=w175) -> ("Micropulse Data"=w176:T42)  [unwired: 7 in, 3 out]
                  n76 = Unbundle By Name(w176) -> ("Command List"=w174:string)
                  n77 = local write "Command List"(w174) -> ()
                }
                event Value Change {
                  w180 = u32 1  # Test No.
                  n78 = event-data() -> ("NewVal"=w184:T13)  [unwired: 1 in, 5 out]
                  n79 = call <instrlib>:"Configure Receive Parameters.vi"("Receive Parameters"=w184, "Test No."=w180) -> ("error out"=w183:errorcluster)  [unwired: 7 in, 2 out]
                  n80 = call <instrlib>:"Read MP Registry Data.vi"("error in (no error)"=w183) -> ("Micropulse Data"=w181:T42)  [unwired: 7 in, 3 out]
                  n81 = Unbundle By Name(w181) -> ("Command List"=w182:string)
                  n82 = local write "Command List"(w182) -> ()
                }
                event Value Change {
                  w185 = u32 1  # Test Number
                  n83 = event-data() -> ("NewVal"=w189:T21)  [unwired: 1 in, 5 out]
                  n84 = call <instrlib>:"Configure Multi Gate Parameters.vi"("Multi Gate Inspection"=w189, "Test Number"=w185) -> ("error out"=w188:errorcluster)  [unwired: 7 in, 2 out]
                  n85 = call <instrlib>:"Read MP Registry Data.vi"("error in (no error)"=w188) -> ("Micropulse Data"=w187:T42)  [unwired: 7 in, 3 out]
                  n86 = Unbundle By Name(w187) -> ("Command List"=w186:string)
                  n87 = local write "Command List"(w186) -> ()
                }
                event Value Change {
                  w190 = u32 1  # Test Number
                  n88 = event-data() -> ()  [unwired: 1 in, 6 out]
                  n89 = local read "Echo Gate Parameters"() -> (w193:T25)
                  n90 = local read "Echo Gate Mode"() -> (w194:T26)
                  n91 = call <instrlib>:"Configure Echo Gate Parameters.vi"("Echo Gate Parameters"=w193, "Echo Trigger Mode"=w194, "Test Number"=w190) -> ("error out"=w195:errorcluster)  [unwired: 6 in, 2 out]
                  n92 = call <instrlib>:"Read MP Registry Data.vi"("error in (no error)"=w195) -> ("Micropulse Data"=w192:T42)  [unwired: 7 in, 3 out]
                  n93 = Unbundle By Name(w192) -> ("Command List"=w191:string)
                  n94 = local write "Command List"(w191) -> ()
                }
                event "Start Acquisition": Value Change {
                  n95 = event-data() -> ()  [unwired: 1 in, 6 out]
                  n96 = call <instrlib>:"Start Continuous Test Cycles [STP].vi"() -> ()  [unwired: 10 in, 2 out]
                }
                event "Stop Acquisition": Value Change {
                  w196 = TRUE  # Erase All? (def F)
                  n97 = event-data() -> ()  [unwired: 1 in, 6 out]
                  n98 = call <instrlib>:"Enter Idle Mode [STX].vi"("Erase All? (def T)"=w196) -> ()  [unwired: 9 in, 2 out]
                }
                event "Acquire Single Scan": Value Change {
                  n99 = event-data() -> ()  [unwired: 1 in, 6 out]
                  n100 = call <instrlib>:"Start 1 Test Cycle [CAL].vi"() -> ()  [unwired: 10 in, 2 out]
                }
                event "A-Scan + Peaks": Scale Range Change {
                  n101 = event-data() -> ()  [unwired: 1 in, 8 out]
                  n102 = call <instrlib>:"Force Gate Update On XY Chart.vi"("Set?"=TRUE, "Test No."=u32 1) -> ()  [unwired: 7 in, 3 out]
                }
                event Value Change {
                  w199 = TRUE
                  # "Stop all activity and reset the hardware to change the sampling frequency"
                  n103 = event-data() -> ()  [unwired: 1 in, 6 out]
                  n104 = local write "Stop"(w199) -> ()
                }
                event Value Change {
                  n105 = event-data() -> ("NewVal"=w201:T27)  [unwired: 1 in, 5 out]
                  n106 = call <instrlib>:"Set Encoder Mode [ENCM].vi"("Encoder Mode"=w201) -> ()  [unwired: 9 in, 2 out]
                }
                event Value Change {
                  n107 = event-data() -> ("NewVal"=w205:T28)  [unwired: 1 in, 5 out]
                  n108 = call <instrlib>:"Set Encoder Settings.vi"("Encoder Settings"=w205, "Axis No."="Axis No.") -> ("error out"=w202:errorcluster)  [unwired: 9 in]
                  n109 = Increment(x="Axis No.") -> (x+1=w203:u8)
                  n110 = call <instrlib>:"Set Encoder Settings.vi"("error in (no error)"=w202, "Encoder Settings"=w205, "Axis No."=w203) -> ()  [unwired: 8 in, 1 out]
                }
                event "Set Position X": Value Change {
                  w206 = u8 1  # Axis No.
                  n111 = event-data() -> ()  [unwired: 1 in, 6 out]
                  n112 = call <instrlib>:"Set Encoder Position [LCP].vi"("Position (mm)"="Position To Set X", "Axis No."=w206) -> ()  [unwired: 8 in, 2 out]
                }
                event "Set Position Y": Value Change {
                  w209 = u8 2  # Axis No.
                  n113 = event-data() -> ()  [unwired: 1 in, 6 out]
                  n114 = call <instrlib>:"Set Encoder Position [LCP].vi"("Position (mm)"="Position To Set Y", "Axis No."=w209) -> ()  [unwired: 8 in, 2 out]
                }
                event Value Change {
                  n115 = event-data() -> ("NewVal"=w211:T3)  [unwired: 1 in, 5 out]
                  n116 = call <instrlib>:"MicroPulse Intensity Colour Tables.vi"("Colour Map Type"=w211) -> ("Colour Table"=w210:u32[])  [unwired: 10 in]
                  n117 = property on="C-Scan Chart" class="IntGraph (strict)"("Color Table"=w210) -> ()  [unwired: 2 in, 2 out]
                  n118 = property on="B-Scan Chart" class="IntGraph (strict)"("Color Table"=w210) -> ()  [unwired: 2 in, 2 out]
                }
                event "Get Status": Value Change {
                  n119 = event-data() -> ()  [unwired: 1 in, 6 out]
                  n120 = call <instrlib>:"Get Status Info [STS].vi"("Request System Status"="Request System Status") -> ()  [unwired: 9 in, 2 out]
                }
                event "Start Test": Value Change {
                  w213 = 0.0 ("Position (mm)")
                  w214 = u8 2  # Axis No.
                  w223 = u8 1  # Axis No.
                  # "Stop any acquisition that's going on"
                  n121 = event-data() -> ()  [unwired: 1 in, 6 out]
                  n122 = call <instrlib>:"Enter Idle Mode [STX].vi"() -> ("error out"=w216:errorcluster)  [unwired: 10 in, 1 out]
                  n123 = call <instrlib>:"FGV-C-Scan Active.vi"("Action"=FGV_-_C-Scan_Active_-_Action_[Enum]."Start C-Scan", "error in (no error)"=w216) -> ("error out"=w215:errorcluster)  [unwired: 7 in, 2 out]
                  n124 = call <instrlib>:"Start Scan (Start to End).vi"("error in (no error)"=w215, "Scan definition"="Axis 1 Scan", "Axis No."=w223) -> ("error out"=w222:errorcluster)  [unwired: 7 in, 1 out]
                  n125 = call <instrlib>:"Set Encoder Position [LCP].vi"("Position (mm)"=w213, "Axis No."=w214) -> ()  [unwired: 8 in, 2 out]
                  n126 = call <instrlib>:"FGV-B-Scan Active.vi"("Action"=FGV_-_B-Scan_Active_-_Action_[Enum]."Start B-Scan", "error in (no error)"=w222) -> ("error out"=w219:errorcluster)  [unwired: 7 in, 2 out]
                  n127 = local write "Position To Set Y"(w213) -> ()
                  n128 = call <instrlib>:"Read MP Registry Data.vi"("error in (no error)"=w219) -> ("Micropulse Data"=w221:T42)  [unwired: 7 in, 3 out]
                  n129 = Unbundle By Name(w221) -> ("Command List"=w220:string)
                  n130 = local write "Command List"(w220) -> ()
                }
                event "Start Free Scan": Value Change {
                  # "use property node so we can sequence starting\nthe B-Scan acitve flags and then enabling the timer"
                  # "Stop any acquisition that's going on"
                  n131 = event-data() -> ()  [unwired: 1 in, 6 out]
                  n132 = call <instrlib>:"Enter Idle Mode [STX].vi"() -> ("error out"=w227:errorcluster)  [unwired: 10 in, 1 out]
                  n133 = call <instrlib>:"FGV-B-Scan Active.vi"("Action"=FGV_-_B-Scan_Active_-_Action_[Enum]."Start B-Scan", "error in (no error)"=w227) -> ("error out"=w226:errorcluster)  [unwired: 7 in, 2 out]
                  n134 = property on="Scan Timer Enabled?" class="Bool (strict)"(error in=w226, "Value"=TRUE ("Scan Timer Enabled?")) -> ()  [unwired: 1 in, 2 out]
                }
                event Key Down {
                  n135 = event-data() -> ("ScanCode"=w229:i16)  [unwired: 1 in, 7 out]
                  n136 = case shown="72" w229 {
                    frame 0, Default {
                    }
                    frame 57 {
                      # "Space bar - Stops all scan activity - returns micropulse to idle mode"
                      # "Space Bar"
                      n137 = call <instrlib>:"FGV-C-Scan Active.vi"() -> ("C-Scan In Progress?"=w230:bool)  [unwired: 9 in, 2 out]
                      n138 = case shown="True" w230 {
                        frame False {
                        }
                        frame True {
                          n139 = call <instrlib>:"Enter Idle Mode [STX].vi"() -> ("error out"=w233:errorcluster)  [unwired: 10 in, 1 out]
                          n140 = call <instrlib>:"FGV-B-Scan Active.vi"("Action"=FGV_-_B-Scan_Active_-_Action_[Enum]."B-Scan Finished", "error in (no error)"=w233) -> ("error out"=w232:errorcluster)  [unwired: 7 in, 2 out]
                          n141 = call <instrlib>:"FGV-C-Scan Active.vi"("Action"=FGV_-_C-Scan_Active_-_Action_[Enum]."C-Scan Finished", "error in (no error)"=w232) -> ()  [unwired: 7 in, 3 out]
                        }
                      }
                    }
                    frame 72 {
                      w237 = u8 2  # Axis No.
                      # "Up Key"
                      n142 = local read "Position To Set Y"() -> (w236:dbl)
                      n143 = Decrement(x=w236) -> (x-1=w235:dbl)
                      n144 = call <instrlib>:"Set Encoder Position [LCP].vi"("Position (mm)"=w235, "Axis No."=w237) -> ()  [unwired: 8 in, 2 out]
                      n145 = local write "Position To Set Y"(w235) -> ()
                    }
                    frame 80 {
                      w240 = u8 2  # Axis No.
                      # "Down Key"
                      n146 = local read "Position To Set Y"() -> (w239:dbl)
                      n147 = Increment(x=w239) -> (x+1=w238:dbl)
                      n148 = call <instrlib>:"Set Encoder Position [LCP].vi"("Position (mm)"=w238, "Axis No."=w240) -> ()  [unwired: 8 in, 2 out]
                      n149 = local write "Position To Set Y"(w238) -> ()
                    }
                  }
                }
                event "Stop C-Scan": Value Change {
                  # "Stops all scan activity - returns micropulse to idle mode."
                  n150 = event-data() -> ()  [unwired: 1 in, 5 out]
                  n151 = call <instrlib>:"FGV-C-Scan Active.vi"() -> ("C-Scan In Progress?"=w243:bool)  [unwired: 9 in, 2 out]
                  n152 = call <instrlib>:"FGV-B-Scan Active.vi"() -> ("B-Scan In Progress?"=w241:bool)  [unwired: 9 in, 2 out]
                  n153 = Or(x=w241, y=w243) -> (x .or. y?=w242:bool)
                  n154 = case shown="True" w242 {
                    frame False {
                    }
                    frame True {
                      n155 = call <instrlib>:"Enter Idle Mode [STX].vi"() -> ("error out"=w246:errorcluster)  [unwired: 10 in, 1 out]
                      n156 = call <instrlib>:"FGV-B-Scan Active.vi"("Action"=FGV_-_B-Scan_Active_-_Action_[Enum]."B-Scan Finished", "error in (no error)"=w246) -> ("error out"=w245:errorcluster)  [unwired: 7 in, 2 out]
                      n157 = call <instrlib>:"FGV-C-Scan Active.vi"("Action"=FGV_-_C-Scan_Active_-_Action_[Enum]."C-Scan Finished", "error in (no error)"=w245) -> ()  [unwired: 7 in, 3 out]
                    }
                  }
                }
                event "Centre Cursor": Value Change {
                  n158 = event-data() -> ()  [unwired: 1 in, 6 out]
                  n159 = property on="B-Scan Chart" class="IntGraph (strict)"() -> ("XScale.Maximum"=w253:dbl, "XScale.Minimum"=w249:dbl)  [unwired: 2 in, 2 out]
                  n160 = Subtract(x=w253, y=w249) -> (x-y=w252:dbl)
                  n161 = Divide(x=w252, y=2.0) -> (x/y=w250:dbl)
                  n162 = Add(x=w250, y=w249) -> (x+y=w248:dbl)
                  n163 = property on="B-Scan Chart" class="IntGraph (strict)"("Cursor.Cursor X"=w248) -> ()  [unwired: 2 in, 2 out]
                }
                event "B-Scan Chart": Cursor Move {
                  n164 = event-data() -> ()  [unwired: 1 in, 8 out]
                  n165 = property on="B-Scan Chart" class="IntGraph (strict)"() -> ("Cursor.Cursor Position"=w254:T47, "Value"=w262:u16[][])  [unwired: 2 in, 2 out]
                  n166 = Unbundle By Name(w254) -> ("Cursor X"=w261:dbl)
                  n167 = property on="A-Scan + Peaks" class="XYGraph (strict)"() -> ("XScale.Multiplier"=w260:dbl, "XScale.Offset"=w259:dbl)  [unwired: 2 in, 2 out]
                  n168 = Index Array(array=w262, index (row)=w261) -> (element=w257:u16[])  [unwired: 1 in]
                  n169 = for {
                    tunnel: w257 -> [_] mode=indexing
                    tunnel: w260 -> [w267]
                    tunnel: w259 -> [w264]
                    tunnel: [w263] -> w258 mode=indexing
                    i -> [w266]
                    n170 = Multiply(x=w267, y=w266) -> (x*y=w265:dbl)
                    n171 = Subtract(x=w265, y=w264) -> (x-y=w263:dbl)
                  }
                  n172 = Bundle(w258, "Value"=w257) -> (w256:cluster{dbl[], "Value":u16[]})  [unwired: 1 in]
                  n173 = Build Array(w256) -> (w255:cluster{dbl[], "Value":u16[]}[])
                  n174 = local write "A-Scan + Peaks"(w255) -> ()
                }
                event Panel Close? {
                  n175 = event-data() -> ()  [unwired: 1 in, 4 out]
                  n176 = event-data("Discard?"=TRUE) -> ()  [unwired: 1 in, 1 out]
                }
                event "QUIT": Value Change {
                  # "set flag to stop acquisition loop"
                  n177 = event-data() -> ()  [unwired: 1 in, 6 out]
                  n178 = call <instrlib>:"FGV-C-Scan Active.vi"("Action"=FGV_-_C-Scan_Active_-_Action_[Enum]."C-Scan Finished") -> ("C-Scan In Progress?"=w270:bool)  [unwired: 8 in, 2 out]
                  n179 = call <instrlib>:"FGV-B-Scan Active.vi"("Action"=FGV_-_B-Scan_Active_-_Action_[Enum]."B-Scan Finished") -> ("B-Scan In Progress?"=w272:bool)  [unwired: 8 in, 2 out]
                  n180 = local write "C-Scan In Progress?"(w270) -> ()
                  n181 = local write "B-Scan In Progress?"(w272) -> ()
                  "Stop" <- TRUE ("Stop")
                }
              }
            }
            n182 = control-ref of="A-Scan + Peaks"() -> (w72:refnum<vi>)
            n183 = property on="B-Scan Chart" class="IntGraph (strict)"() -> ("Plot Area Size"=w69:T48)  [unwired: 2 in, 2 out]
            n184 = while {
              tunnel: w72 -> [w99]
              tunnel: [w98] -> w71
              tunnel: w69 -> [w89]
              stop <- w97 stop-if-true
              w96 = u8 1  # Axis No.
              # "Asynchronous Read from Micropulse"
              n185 = call <instrlib>:"Read MP Message.vi"() -> ("error out"=w100:errorcluster, "scan data info"=w93:T49, "Instrument Message"=w103:string)  [unwired: 7 in, 2 out]
              n186 = call <instrlib>:"Instrument Message History.vi"("Instrument Message"=w103) -> ("Message Count"=→"message count":i32, "Message History out"=→"System Messages":string)  [unwired: 9 in]
              n187 = Unbundle By Name(w93) -> ("Test No."=w101:u32)
              n188 = case shown="1" w101 {
                selector: w101 -> [_ w120]
                tunnel: w93 -> [_ w113]
                tunnel: w100 -> [w106 w122]
                tunnel: w99 -> [_ w119]
                tunnel: [w106 w121] -> w98
                tunnel: w89 -> [_ w107]
                frame -1, Default {
                }
                frame 1 {
                  # "To save CPU time and allow for updates due to cursor moves, we restrict unnecessary updates from the uPulse to live data."
                  n189 = local read "Axis No."() -> (w115:u8)
                  n190 = call <instrlib>:"AScan+Peaks to XY Chart.vi"("error in (no error)"=w122, "scan data info"=w113, "Test No."=w120) -> ("error out"=w123:errorcluster, "Echo Range (us)"=w118:dbl, "AScan+Peaks"=w126:cluster{"timebase":dbl[], "data":u16[]}[], "Update Indicators?"=w109:bool, "Running Average PRF"=→"running average PRF":dbl)  [unwired: 3 in, 1 out]
                  n191 = case shown="\"Absolute Scan [FLX+FLZ]\", Default" "Scan Choice" {
                    tunnel: [w140 _] -> w117
                    tunnel: [w146 w156] -> w111
                    tunnel: w115 -> [w148 _]
                    tunnel: [w142 w153] -> w108
                    tunnel: w113 -> [w149 w155]
                    tunnel: [w147 u16[][] [] ("C-Scan Out")] -> w112
                    tunnel: [w145 FALSE ("C-Scan In Progress?")] -> w110
                    frame "Absolute Scan [FLX+FLZ]", Default {
                      n192 = local read "Axis 2 Scan"() -> (w144:T31)
                      n193 = local read "Axis 1 Scan"() -> (w143:T30)
                      n194 = call <instrlib>:"C-Scan (LLC messages).vi"("Define C-Scan Index"=w144, "Scan definition"=w143, "Axis No."=w148, "scan data info"=w149) -> ("C-Scan In Progress?"=w145:bool, "C-Scan Out"=w147:u16[][])  [unwired: 4 in, 2 out]
                      n195 = call <instrlib>:"B-Scan (LLC messages) DVR.vi"("Scan definition"=w143, "Axis No."=w148, "scan data info"=w149) -> ("Update Display?"=w150:bool, "B-Scan In Progress?"=w146:bool, "data value reference"=w140:refnum<data-value>)  [unwired: 5 in, 1 out]
                      n196 = call <instrlib>:"C-Scan - Reverse B-Scan.vi"("FLZ Scan definition"=w143, "C-Scan In Progress?"=w145, "B-Scan In Progress?"=w146) -> ("B-Scan Just Finished?"=w141:bool)  [unwired: 8 in]
                      n197 = Or(x=w150, y=w141) -> (x .or. y?=w142:bool)
                    }
                    frame "Free Scan" {
                      n198 = local read "Scan definition"() -> (w154:T1)
                      n199 = call <instrlib>:"B-Scan (Timed) DVR.vi"("Scan definition"=w154, "scan data info"=w155) -> ("Update Display?"=w153:bool, "B-Scan In Progress?"=w156:bool)  [unwired: 6 in, 2 out]
                    }
                  }
                  "B-Scan In Progress?" <- w111
                  "C-Scan In Progress?" <- w110
                  n200 = Index Array(array=w126, index="Gate No.") -> (element=→"peak data":cluster{"timebase":dbl[], "data":u16[]})
                  n201 = case shown="True" w109 {
                    tunnel: w126 -> [_ w134]
                    tunnel: w123 -> [w127 w132]
                    tunnel: [w127 w131] -> w121
                    tunnel: w120 -> [_ w130]
                    tunnel: w119 -> [_ w129]
                    tunnel: w118 -> [_ w128]
                    frame False {
                    }
                    frame True {
                      n202 = call <instrlib>:"Adjust Peak Offsets On XY Chart.vi"("error in (no error)"=w132, "Echo Range in"=w128, "AScan+Peaks in"=w134) -> ("error out"=w133:errorcluster, "AScan+Peaks out"=→"A-Scan + Peaks":cluster{"timebase":dbl[], "data":u16[]}[])  [unwired: 7 in]
                      n203 = call <instrlib>:"Draw Gates On XY Chart.vi"("error in (no error)"=w133, "Echo Range"=w128, "XYGraph in"=w129, "Test No."=w130) -> ("error out"=w131:errorcluster)  [unwired: 7 in]
                    }
                  }
                  "live error out" <- w121
                  n204 = case shown="True" w108 {
                    tunnel: w117 -> [_ w136]
                    tunnel: w112 -> [_ w139]
                    tunnel: w107 -> [_ w138]
                    frame False {
                    }
                    frame True {
                      n205 = call <instrlib>:"Decimate Data For 2D Intensity Chart - DVR.vi"("Plot Area"=w138, "data value reference"=w136) -> ("Decimated Display"=→"B-Scan Chart":u16[][])  [unwired: 9 in]
                      "C-Scan Chart" <- w139
                    }
                  }
                }
              }
              n206 = Unbundle By Name(w93) -> ("Axis Positions.Axis 1"=w95:u32, "Axis Positions.Axis 2"=w92:u32)
              n207 = call <instrlib>:"Get Abolute Location From Inspection Point (1-Ch).vi"("Inspection Point Location"=w95, "Axis No."=w96) -> ("Absolute Location"=→"X Current Position":dbl)  [unwired: 9 in]
              n208 = call <instrlib>:"Get Abolute Location From Inspection Point (1-Ch).vi"("Inspection Point Location"=w92, "Axis No."=u8 2) -> ("Absolute Location"=→"Y Current Position":dbl)  [unwired: 9 in]
              n209 = flat-sequence {
                tunnel: [w105] -> w97
                tunnel: w98 -> [_]
                frame #0 {
                  n210 = local read "Stop"() -> (w105:bool)
                }
              }
            }
          }
          frame Error {
          }
        }
        n211 = Select(t=Main_Program_State_-_Enum."Reset HW", s=w64, f=Main_Program_State_-_Enum."Shutdown") -> (s? t:f=w63:T38)
      }
      frame "Reset HW" {
        # "Close the connection to allow for reopening in the \"Init HW\" case"
        n212 = call <instrlib>:"Close.vi"("error in (no error)"=w279) -> ("error out"=w278:errorcluster)  [unwired: 9 in, 1 out]
      }
      frame "Shutdown" {
        # "Terminate the TCP/IP connection"
        n213 = local write "Stop"(FALSE ("stop")) -> ()
        n214 = call <instrlib>:"Close.vi"() -> ()  [unwired: 10 in, 2 out]
      }
    }
  }
